vi "PROCESSADOR_bat_PC2.vi"() -> ()   [LabVIEW 2019]
uses:
  <vilib>/Utility/file.llb/Read Delimited Spreadsheet (string).vi
panel:
  out "Numeric":i32
  in  "Previstas":i32=37200
  out "Grupos iter":i32
  out "Freqs iter":i32
  in  "Frequências?":bool=TRUE
  out "Frequência":string
  out "Simulando:":string
  in  "Auto":bool=TRUE
  in  "Ger. Distr.":bool
  in  "Y ? ou D":bool
  in  "Eq. + Trafo":bool=TRUE
  in  "Linhas acopladas":bool=TRUE
  in  "Carga mista":bool=TRUE
  out "path":path
  in  "numera\narquivos":bool
  out "Previstas":i32
  out "Loads (out)":string[](array[string])
  out "inicial":i32
  in  "run minimized? (F)":bool=TRUE
  out "Simulando?":bool
  out "Em processo":i32
  out "Processadas":i32
  out "minutos":dbl
  out "horas":dbl
  out "Elapsed Time (s)":dbl
  in  "Endereço de saída (.atp)":path=path "C:/DADOS/arquivos_atp"
  out "Restantes":i32
  in  "simular?":bool=TRUE
  in  "Endereço de saída (.mat)":path=path "C:/DADOS/Eventos"
  in  "Lista de condições (arquivo.txt)":string="lista_condicoes_CARGAS.txt"
  in  "Diretório de trabalho":path=path "C:/ATP/ATPDraw/Projects_Flavio"
  out "Casos":string[][](array[string])
  # "ATPmanager - Gerenciador de simulações"
  # "*Configurado para operar em conjunto com MATLAB - v2"
  # "Simulações"
  # "________________________________________________________________________"
  # "(trafo com bug - \nusando imped eq)"
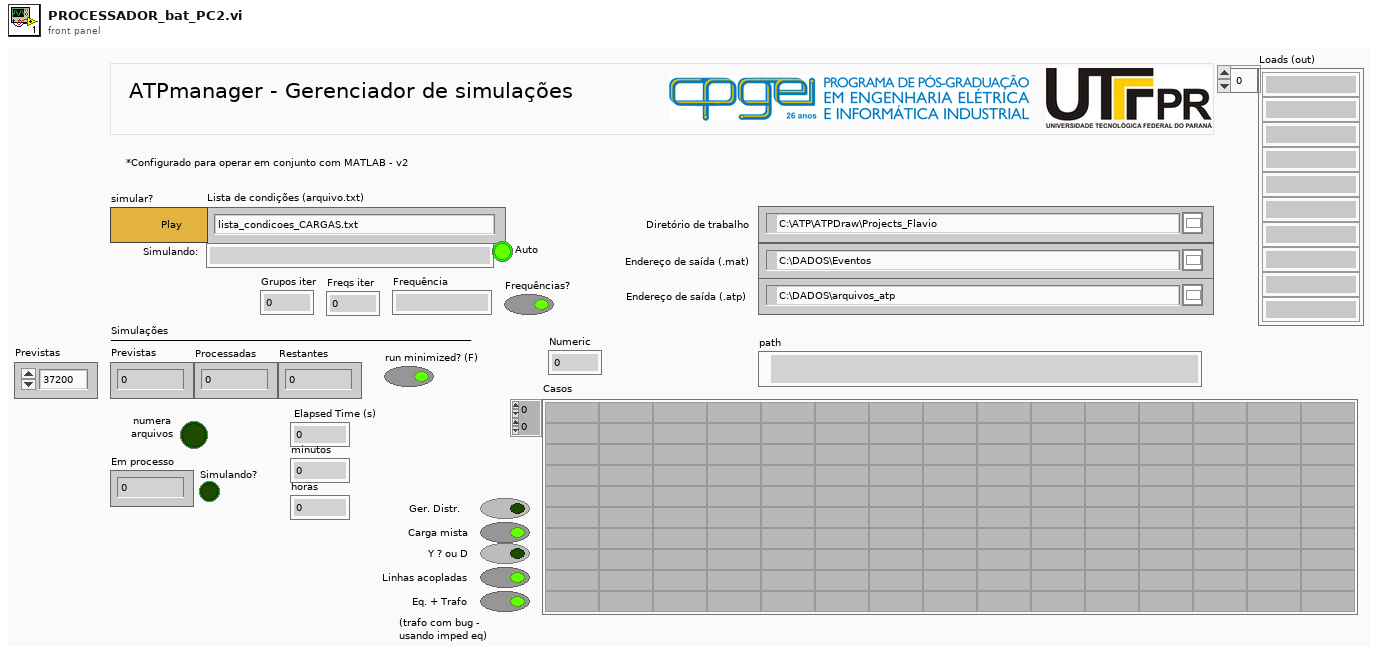
[diagram p1: front panel]
types:
  T1 = cluster{"Ger. Distr.":bool, "Carga mista":bool, "Linhas acopladas":bool, "Eq. + Trafo":bool, "Y ? ou D":bool}
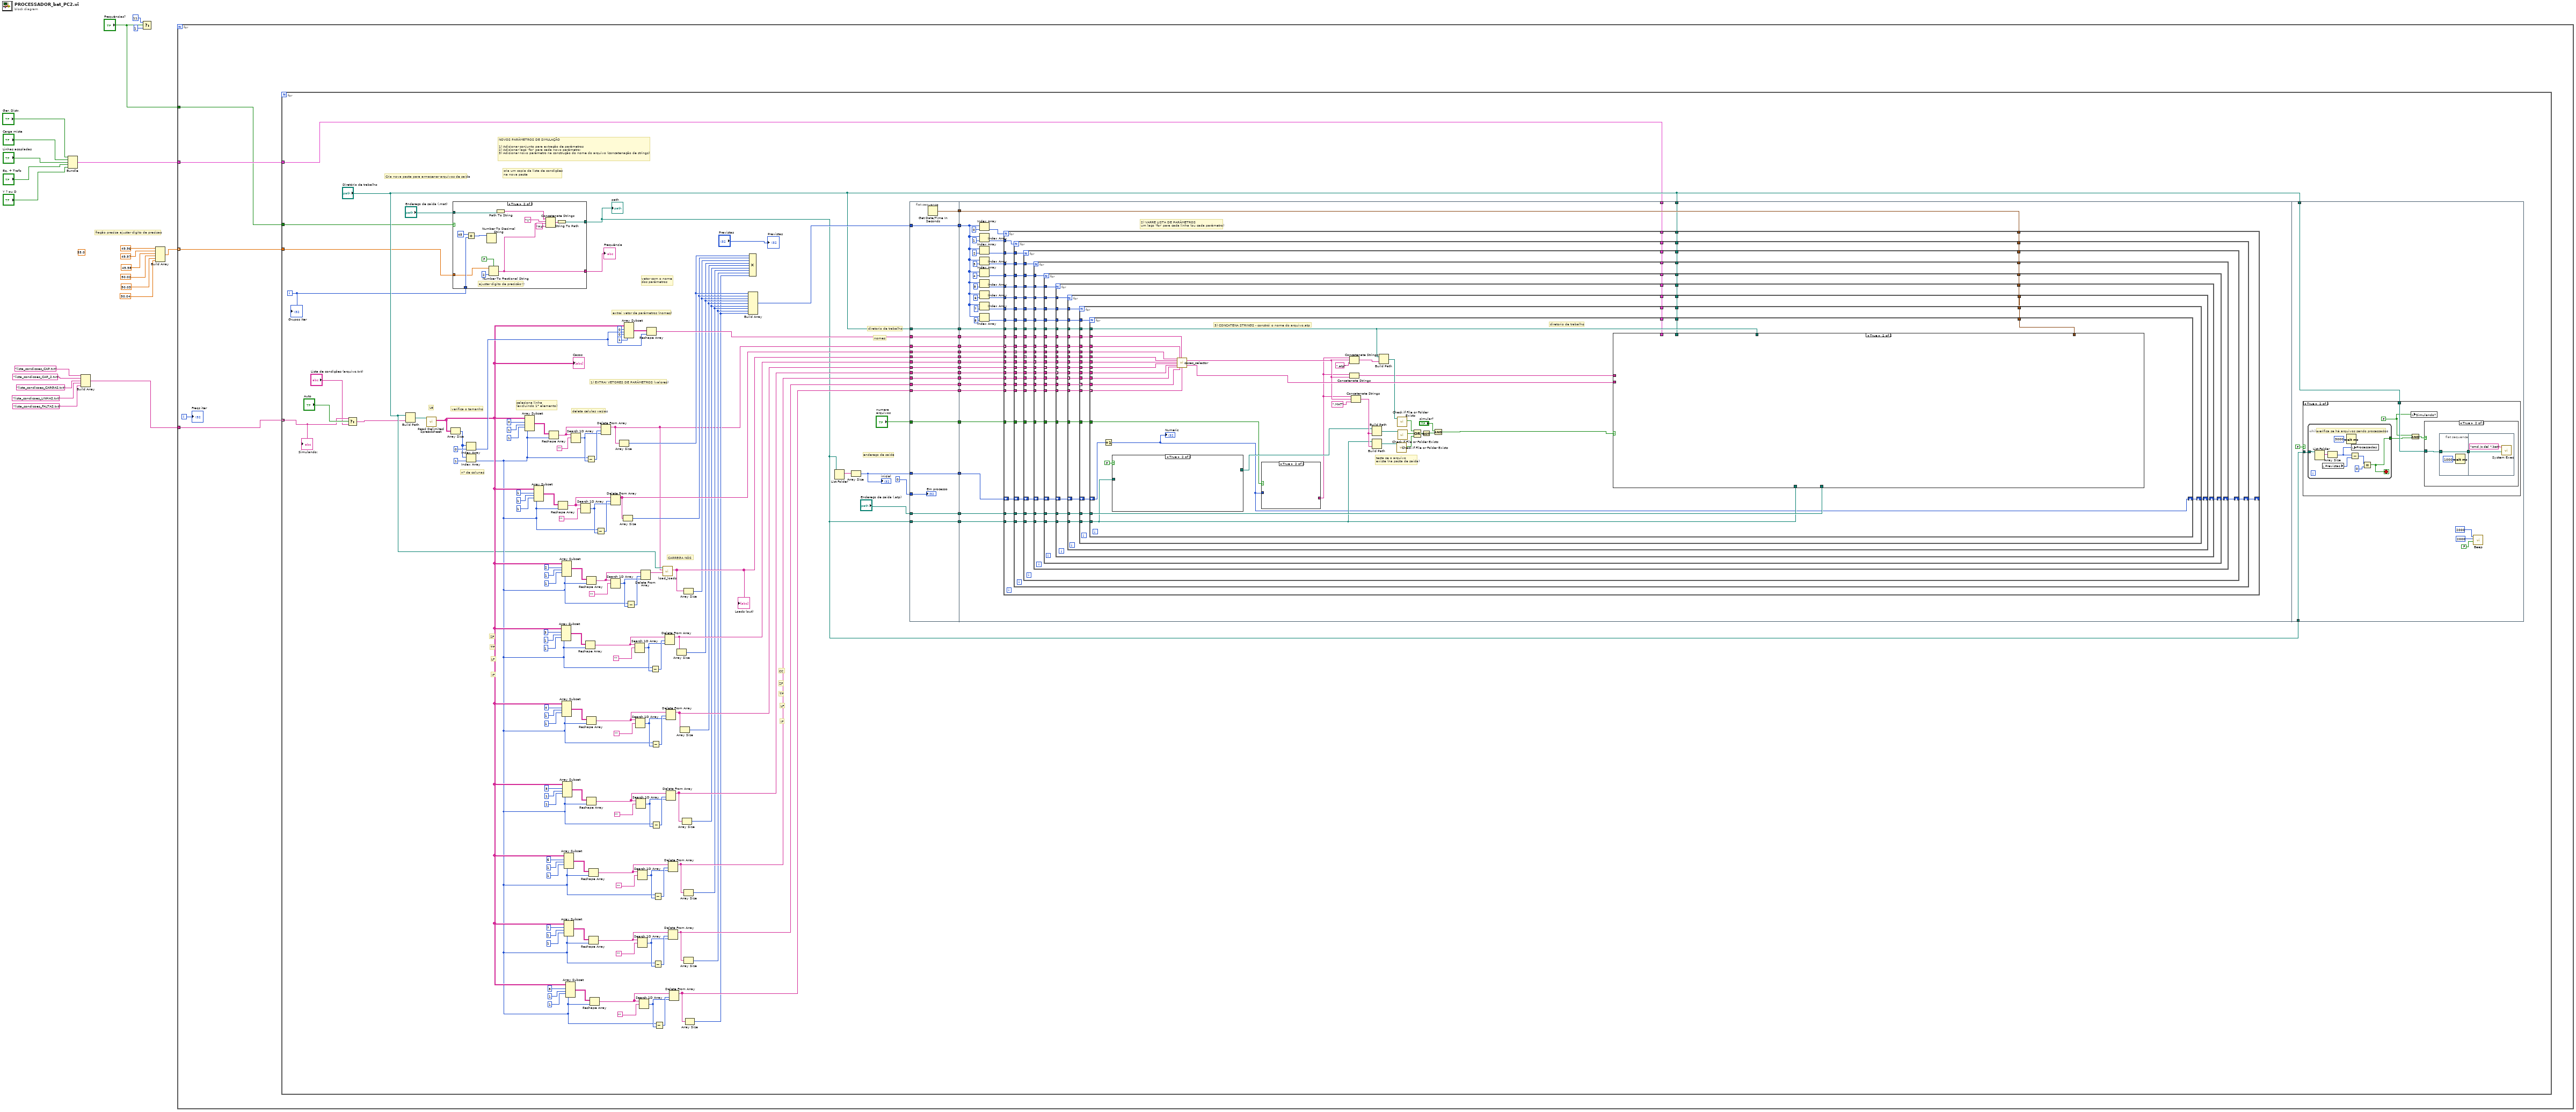
[diagram p0: block diagram]
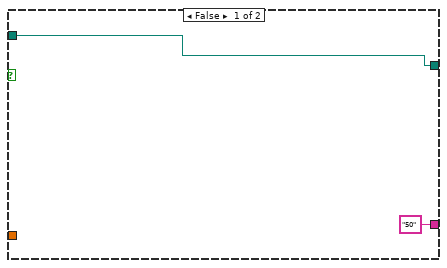
[diagram p2: hidden frame]
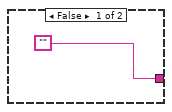
[diagram p4: hidden frame]
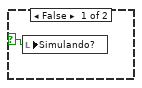
[diagram p5: hidden frame]
diagram:
  (unwired) 55.0
  # "fração precisa ajustar digito de precisao"
  n1 = Bundle("Ger. Distr."="Ger. Distr.", "Carga mista"="Carga mista", "Linhas acopladas"="Linhas acopladas", "Eq. + Trafo"="Eq. + Trafo", "Y ? ou D"="Y ? ou D") -> (w18:T1)  [unwired: 1 in]
  n2 = Build Array("lista_condicoes_CAP.txt", "lista_condicoes_CAP_2.txt", "lista_condicoes_CARGAS.txt", "lista_condicoes_LINHAS.txt", "lista_condicoes_FALTAS.txt") -> (w12:string[])
  n3 = Select(t=11, s="Frequências?", f=1) -> ()  [unwired: 1 out]
  n4 = Build Array(49.96, 49.97, 49.98, 50.02, 50.03, 50.04) -> (w16:dbl[])
  n5 = for {
    tunnel: w18 -> [w27]
    tunnel: w12 -> [w26]
    tunnel: w16 -> [w25] mode=indexing
    tunnel: "Frequências?" -> [w24]
    i -> [w23]
    n6 = for {
      tunnel: w24 -> [w37]
      tunnel: w27 -> [w35]
      tunnel: w26 -> [w32] mode=indexing
      tunnel: w25 -> [w30]
      i -> [w36]
      # "CARREGA NÓS"
      # "deleta celulas vazias"
      # "seleciona linha\n(excluindo 1° elemento)"
      # "endereço de saída"
      # "nomes"
      # "diretorio de trabalho"
      # "LF"
      # "TF"
      # "IF"
      # "ZF"
      # "CC"
      # "LF"
      # "TF"
      # "IF"
      # "ZF"
      # "cria um copia da lista de condições\nna nova pasta"
      # "Cria nova pasta para armazenar arquivos de saída"
      # "extrai vetor de parâmetros (nomes)"
      # "1) EXTRAI VETORES DE PARÂMETROS (valores)"
      # "NOVOS PARÂMETROS DE SIMULAÇÃO\n\n1) Adicionar conjunto para extração de parâmetros\n2) Adicionar laço 'for' para cada novo parâmetro;\n3) Adicionar novo parâmetro na construção do nome do arquivo (concatenação de strings)"
      # "vetor com o nome\ndos parâmetros"
      # "n° de colunas"
      # "verifica o tamanho"
      # "Lê"
      n7 = Select(t=w32, s="Auto", f="Lista de condições (arquivo.txt)") -> (s? t:f=w34:string)
      n8 = Build Path(base path="Diretório de trabalho", name or relative path=w34) -> (appended path=w98:path)
      n9 = call-poly <vilib>:"Read Delimited Spreadsheet.vi"("file path (dialog if empty)"=w98) -> ("all rows"=w59:string[][])  [unwired: 9 in, 5 out]
      "Casos" <- w59
      n10 = Array Size(array=w59) -> (size(s)=w147:i32[])
      n11 = case shown="True" w37 {
        tunnel: [w168 w181] -> w39
        tunnel: "Endereço de saída (.mat)" -> [w168 w179]
        tunnel: w36 -> [_ w175]
        tunnel: w30 -> [_ w170]
        tunnel: ["50" w169] -> w28
        frame False {
        }
        frame True {
          # "ajustar digito de precisão!!!"
          n12 = Add(x=45, y=w175) -> (x+y=w173:i32)
          n13 = Number To Decimal String(number=w173) -> ()  [unwired: 1 in, 1 out]
          n14 = Number To Fractional String(use system decimal point (T)=FALSE, number=w170, precision (6)=i16 2) -> (F-format string=w169:string)  [unwired: 1 in]
          n15 = Path To String(path=w179) -> (string=w178:string)
          n16 = Concatenate Strings(w178, "\\" ("string"), w169, "Hz" ("string")) -> (w180:string)
          n17 = String To Path(string=w180) -> (path=w181:path)
        }
      }
      "path" <- w39
      "Frequência" <- w28
      n18 = Index Array(array=w147, index=0) -> (element=w97:i32)
      n19 = Index Array(array=w147, index=1) -> (element=w58:i32)
      n20 = Array Subset(array=w59, index (row)=0 ("index"), length (row)=1 ("length"), index (col)=1 ("index"), length (col)=w58) -> (w93:string[][])
      n21 = Array Subset(array=w59, index (row)=1 ("index"), length (row)=1 ("length"), index (col)=1 ("index"), length (col)=w58) -> (w139:string[][])
      n22 = Reshape Array(w93, w58) -> (w91:string[])
      n23 = Reshape Array(w139, w58) -> (w137:string[])
      n24 = Array Subset(array=w59, index (row)=3 ("index"), length (row)=1 ("length"), index (col)=1 ("index"), length (col)=w58) -> (w123:string[][])
      n25 = Array Subset(array=w59, index (row)=2 ("index"), length (row)=1 ("length"), index (col)=1 ("index"), length (col)=w58) -> (w131:string[][])
      n26 = Array Subset(array=w59, index (row)=4 ("index"), length (row)=1 ("length"), index (col)=1 ("index"), length (col)=w58) -> (w115:string[][])
      n27 = Array Subset(array=w59, index (row)=5 ("index"), length (row)=1 ("length"), index (col)=1 ("index"), length (col)=w58) -> (w107:string[][])
      n28 = Array Subset(array=w59, index (row)=6 ("index"), length (row)=1 ("length"), index (col)=1 ("index"), length (col)=w58) -> (w80:string[][])
      n29 = Array Subset(array=w59, index (row)=7 ("index"), length (row)=1 ("length"), index (col)=1 ("index"), length (col)=w58) -> (w72:string[][])
      n30 = Array Subset(array=w59, index (row)=8 ("index"), length (row)=1 ("length"), index (col)=1 ("index"), length (col)=w58) -> (w64:string[][])
      n31 = Search 1D Array(1D array=w91, element="") -> (index of element=w89:i32)  [unwired: 1 in]
      n32 = Search 1D Array(1D array=w137, element="") -> (index of element=w135:i32)  [unwired: 1 in]
      n33 = Reshape Array(w123, w58) -> (w121:string[])
      n34 = Subtract(x=w58, y=w89) -> (x-y=w90:i32)
      n35 = Reshape Array(w131, w58) -> (w129:string[])
      n36 = Reshape Array(w115, w58) -> (w113:string[])
      n37 = Reshape Array(w107, w58) -> (w105:string[])
      n38 = Reshape Array(w80, w58) -> (w78:string[])
      n39 = Reshape Array(w72, w58) -> (w70:string[])
      n40 = Reshape Array(w64, w58) -> (w62:string[])
      n41 = Subtract(x=w58, y=w135) -> (x-y=w136:i32)
      n42 = Delete From Array(array=w91, length=w90, index=w89) -> (array with subset deleted=w41:string[])  [unwired: 1 out]
      n43 = Delete From Array(array=w137, length=w136, index=w135) -> (array with subset deleted=w87:string[])  [unwired: 1 out]
      n44 = Search 1D Array(1D array=w129, element="") -> (index of element=w127:i32)  [unwired: 1 in]
      n45 = Array Size(array=w41) -> (size(s)=w50:i32)
      n46 = Array Size(array=w87) -> (size(s)=w49:i32)
      n47 = Array Subset(array=w59, index (row)=0 ("index"), length (row)=w97, index (col)=0 ("index"), length (col)=1 ("length")) -> (w143:string[][])
      n48 = Subtract(x=w58, y=w127) -> (x-y=w128:i32)
      n49 = Search 1D Array(1D array=w121, element="") -> (index of element=w119:i32)  [unwired: 1 in]
      n50 = Search 1D Array(1D array=w113, element="") -> (index of element=w111:i32)  [unwired: 1 in]
      n51 = Search 1D Array(1D array=w105, element="") -> (index of element=w103:i32)  [unwired: 1 in]
      n52 = Search 1D Array(1D array=w78, element="") -> (index of element=w76:i32)  [unwired: 1 in]
      n53 = Search 1D Array(1D array=w70, element="") -> (index of element=w68:i32)  [unwired: 1 in]
      n54 = Search 1D Array(1D array=w62, element="") -> (index of element=w60:i32)  [unwired: 1 in]
      n55 = Delete From Array(array=w129, length=w128, index=w127) -> (array with subset deleted=w53:string[])  [unwired: 1 out]
      n56 = Reshape Array(w143, w97) -> (w96:string[])
      n57 = Subtract(x=w58, y=w119) -> (x-y=w120:i32)
      n58 = Subtract(x=w58, y=w111) -> (x-y=w112:i32)
      n59 = Subtract(x=w58, y=w103) -> (x-y=w104:i32)
      n60 = Subtract(x=w58, y=w76) -> (x-y=w77:i32)
      n61 = Subtract(x=w58, y=w68) -> (x-y=w69:i32)
      n62 = Subtract(x=w58, y=w60) -> (x-y=w61:i32)
      n63 = call "load_loads.vi"("Nodes"=w53, "Events"=w41, "Diretório de trabalho"="Diretório de trabalho") -> ("Loads (out)"=w51:string[])  [unwired: 8 in]
      "Loads (out)" <- w51
      n64 = Delete From Array(array=w121, length=w120, index=w119) -> (array with subset deleted=w86:string[])  [unwired: 1 out]
      n65 = Delete From Array(array=w113, length=w112, index=w111) -> (array with subset deleted=w85:string[])  [unwired: 1 out]
      n66 = Delete From Array(array=w105, length=w104, index=w103) -> (array with subset deleted=w84:string[])  [unwired: 1 out]
      n67 = Delete From Array(array=w78, length=w77, index=w76) -> (array with subset deleted=w57:string[])  [unwired: 1 out]
      n68 = Delete From Array(array=w70, length=w69, index=w68) -> (array with subset deleted=w56:string[])  [unwired: 1 out]
      n69 = Delete From Array(array=w62, length=w61, index=w60) -> (array with subset deleted=w55:string[])  [unwired: 1 out]
      n70 = Array Size(array=w86) -> (size(s)=w47:i32)
      n71 = Array Size(array=w85) -> (size(s)=w46:i32)
      n72 = Array Size(array=w84) -> (size(s)=w45:i32)
      n73 = Array Size(array=w51) -> (size(s)=w48:i32)
      n74 = Array Size(array=w57) -> (size(s)=w44:i32)
      n75 = Array Size(array=w56) -> (size(s)=w43:i32)
      n76 = Array Size(array=w55) -> (size(s)=w42:i32)
      n77 = Build Array(w50, w49, w48, w47, w46, w45, w44, w43, w42) -> (w54:i32[])
      n78 = Compound Arithmetic op=MULTIPLY(w50, w49, w48, w47, w46, w45, w44, w43, w42) -> ()  [unwired: 1 out]
      n79 = List Folder(path=w39) -> (filenames=w100:string[])  [unwired: 3 in, 3 out]
      n80 = Array Size(array=w100) -> (size(s)=w99:i32)
      "inicial" <- w99
      n81 = flat-sequence {
        tunnel: w96 -> [w198]
        tunnel: "Diretório de trabalho" -> [w199]
        tunnel: [w199] -> w166
        tunnel: [w198] -> w165
        tunnel: [w197] -> w164
        tunnel: "Endereço de saída (.atp)" -> [w197]
        tunnel: [w196] -> w163
        tunnel: [w193] -> w162
        tunnel: 0 -> [w195]
        tunnel: w39 -> [w194]
        tunnel: [w194] -> w161
        tunnel: w99 -> [w193]
        tunnel: w54 -> [w192]
        tunnel: [w192] -> w160
        tunnel: w41 -> [w191]
        tunnel: [w191] -> w159
        tunnel: w87 -> [w190]
        tunnel: w51 -> [w189]
        tunnel: w86 -> [w188]
        tunnel: w85 -> [w187]
        tunnel: w84 -> [w186]
        tunnel: [w190] -> w158
        tunnel: [w189] -> w157
        tunnel: [w188] -> w156
        tunnel: [w187] -> w155
        tunnel: [w186] -> w154
        tunnel: [w185] -> w153
        tunnel: w57 -> [w185]
        tunnel: [w184] -> w152
        tunnel: w56 -> [w184]
        tunnel: [w183] -> w151
        tunnel: w55 -> [w183]
        tunnel: [w182] -> w150
        tunnel: "numera\narquivos" -> [w182]
        tunnel: w166 -> [w236]
        tunnel: w165 -> [w235]
        tunnel: w164 -> [w234]
        tunnel: w163 -> [w233]
        tunnel: w162 -> [w230]
        tunnel: w161 -> [w232]
        tunnel: "Diretório de trabalho" -> [w231]
        tunnel: w160 -> [w220]
        tunnel: w159 -> [w210]
        tunnel: w158 -> [w209]
        tunnel: w157 -> [w208]
        tunnel: w156 -> [w207]
        tunnel: w155 -> [w206]
        tunnel: w154 -> [w205]
        tunnel: w153 -> [w204]
        tunnel: w152 -> [w203]
        tunnel: w151 -> [w202]
        tunnel: w150 -> [w201]
        tunnel: w35 -> [w200]
        tunnel: "Diretório de trabalho" -> [w540]
        tunnel: w39 -> [w541]
        frame #0 {
          n82 = Get Date/Time In Seconds() -> (seconds since 1Jan1904=w196:timestamp)
          "Em processo" <- w195
        }
        frame #1 {
          # "2) VARRE LISTA DE PARÂMETROS\num laço 'for' para cada linha (ou cada parâmetro)"
          n83 = Index Array(array=w220, index=0) -> (element=w219:i32)
          n84 = Index Array(array=w220, index=1) -> (element=w218:i32)
          n85 = Index Array(array=w220, index=2) -> (element=w217:i32)
          n86 = Index Array(array=w220, index=3) -> (element=w216:i32)
          n87 = Index Array(array=w220, index=4) -> (element=w215:i32)
          n88 = Index Array(array=w220, index=5) -> (element=w214:i32)
          n89 = Index Array(array=w220, index=6) -> (element=w213:i32)
          n90 = Index Array(array=w220, index=7) -> (element=w212:i32)
          n91 = Index Array(array=w220, index=8) -> (element=w211:i32)
          n92 = for {
            N: w219 -> [_]
            tunnel: w236 -> [w263]
            tunnel: w235 -> [w262]
            tunnel: w234 -> [w261]
            tunnel: w233 -> [w260]
            tunnel: w232 -> [w258]
            tunnel: w231 -> [w257]
            shift-right: [w259] -> _
            shift-left: w230 -> [w256]
            tunnel: w218 -> [w255]
            tunnel: w217 -> [w254]
            tunnel: w216 -> [w253]
            tunnel: w215 -> [w252]
            tunnel: w214 -> [w251]
            tunnel: w213 -> [w250]
            tunnel: w212 -> [w249]
            tunnel: w211 -> [w248]
            tunnel: w210 -> [w247] mode=indexing
            tunnel: w209 -> [w246]
            tunnel: w208 -> [w245]
            tunnel: w207 -> [w244]
            tunnel: w206 -> [w243]
            tunnel: w205 -> [w242]
            tunnel: w204 -> [w241]
            tunnel: w203 -> [w240]
            tunnel: w202 -> [w239]
            tunnel: w201 -> [w238]
            tunnel: w200 -> [w237]
            n93 = for {
              N: w255 -> [_]
              tunnel: w263 -> [w289]
              tunnel: w262 -> [w288]
              tunnel: w261 -> [w287]
              tunnel: w260 -> [w286]
              tunnel: w258 -> [w284]
              tunnel: w257 -> [w283]
              shift-right: [w285] -> w259
              shift-left: w256 -> [w282]
              tunnel: w254 -> [w281]
              tunnel: w253 -> [w280]
              tunnel: w252 -> [w279]
              tunnel: w251 -> [w278]
              tunnel: w250 -> [w277]
              tunnel: w249 -> [w276]
              tunnel: w248 -> [w275]
              tunnel: w247 -> [w274]
              tunnel: w246 -> [w273] mode=indexing
              tunnel: w245 -> [w272]
              tunnel: w244 -> [w271]
              tunnel: w243 -> [w270]
              tunnel: w242 -> [w269]
              tunnel: w241 -> [w268]
              tunnel: w240 -> [w267]
              tunnel: w239 -> [w266]
              tunnel: w238 -> [w265]
              tunnel: w237 -> [w264]
              n94 = for {
                N: w281 -> [_]
                tunnel: w289 -> [w314]
                tunnel: w288 -> [w313]
                tunnel: w287 -> [w312]
                tunnel: w286 -> [w311]
                tunnel: w284 -> [w309]
                tunnel: w283 -> [w308]
                shift-right: [w310] -> w285
                shift-left: w282 -> [w307]
                tunnel: w280 -> [w306]
                tunnel: w279 -> [w305]
                tunnel: w278 -> [w304]
                tunnel: w277 -> [w303]
                tunnel: w276 -> [w302]
                tunnel: w275 -> [w301]
                tunnel: w274 -> [w300]
                tunnel: w273 -> [w299]
                tunnel: w272 -> [w298] mode=indexing
                tunnel: w271 -> [w297]
                tunnel: w270 -> [w296]
                tunnel: w269 -> [w295]
                tunnel: w268 -> [w294]
                tunnel: w267 -> [w293]
                tunnel: w266 -> [w292]
                tunnel: w265 -> [w291]
                tunnel: w264 -> [w290]
                n95 = for {
                  N: w306 -> [_]
                  tunnel: w314 -> [w338]
                  tunnel: w313 -> [w337]
                  shift-right: [w336] -> w310
                  shift-left: w307 -> [w333]
                  tunnel: w312 -> [w335]
                  tunnel: w311 -> [w334]
                  tunnel: w309 -> [w332]
                  tunnel: w308 -> [w331]
                  tunnel: w305 -> [w329]
                  tunnel: w304 -> [w330]
                  tunnel: w303 -> [w328]
                  tunnel: w302 -> [w327]
                  tunnel: w301 -> [w326]
                  tunnel: w300 -> [w325]
                  tunnel: w299 -> [w324]
                  tunnel: w298 -> [w323]
                  tunnel: w297 -> [w322] mode=indexing
                  tunnel: w296 -> [w321]
                  tunnel: w295 -> [w320]
                  tunnel: w294 -> [w319]
                  tunnel: w293 -> [w318]
                  tunnel: w292 -> [w317]
                  tunnel: w291 -> [w316]
                  tunnel: w290 -> [w315]
                  n96 = for {
                    N: w329 -> [_]
                    tunnel: w337 -> [w361]
                    tunnel: w338 -> [w360]
                    shift-right: [w358] -> w336
                    shift-left: w333 -> [w359]
                    tunnel: w335 -> [w357]
                    tunnel: w334 -> [w356]
                    tunnel: w332 -> [w355]
                    tunnel: w331 -> [w354]
                    tunnel: w330 -> [w353]
                    tunnel: w328 -> [w352]
                    tunnel: w327 -> [w351]
                    tunnel: w326 -> [w350]
                    tunnel: w325 -> [w349]
                    tunnel: w324 -> [w348]
                    tunnel: w323 -> [w347]
                    tunnel: w322 -> [w346]
                    tunnel: w321 -> [w344] mode=indexing
                    tunnel: w320 -> [w345]
                    tunnel: w319 -> [w343]
                    tunnel: w318 -> [w342]
                    tunnel: w317 -> [w341]
                    tunnel: w316 -> [w340]
                    tunnel: w315 -> [w339]
                    n97 = for {
                      N: w353 -> [_]
                      tunnel: w361 -> [w383]
                      tunnel: w360 -> [w382]
                      shift-right: [w380] -> w358
                      shift-left: w359 -> [w381]
                      tunnel: w357 -> [w379]
                      tunnel: w356 -> [w378]
                      tunnel: w355 -> [w377]
                      tunnel: w354 -> [w376]
                      tunnel: w352 -> [w375]
                      tunnel: w351 -> [w374]
                      tunnel: w350 -> [w373]
                      tunnel: w349 -> [w372]
                      tunnel: w348 -> [w371]
                      tunnel: w347 -> [w370]
                      tunnel: w346 -> [w369]
                      tunnel: w345 -> [w368] mode=indexing
                      tunnel: w344 -> [w367]
                      tunnel: w343 -> [w366]
                      tunnel: w342 -> [w365]
                      tunnel: w341 -> [w364]
                      tunnel: w340 -> [w363]
                      tunnel: w339 -> [w362]
                      n98 = for {
                        N: w375 -> [_]
                        tunnel: w383 -> [w404]
                        tunnel: w382 -> [w403]
                        shift-right: [w401] -> w380
                        shift-left: w381 -> [w402]
                        tunnel: w379 -> [w400]
                        tunnel: w378 -> [w399]
                        tunnel: w377 -> [w398]
                        tunnel: w376 -> [w397]
                        tunnel: w374 -> [w396]
                        tunnel: w373 -> [w395]
                        tunnel: w372 -> [w394]
                        tunnel: w371 -> [w393]
                        tunnel: w370 -> [w392]
                        tunnel: w369 -> [w391]
                        tunnel: w368 -> [w390]
                        tunnel: w367 -> [w389]
                        tunnel: w366 -> [w388] mode=indexing
                        tunnel: w365 -> [w387]
                        tunnel: w364 -> [w386]
                        tunnel: w363 -> [w385]
                        tunnel: w362 -> [w384]
                        n99 = for {
                          N: w396 -> [_]
                          tunnel: w404 -> [w424]
                          tunnel: w403 -> [w423]
                          shift-right: [w421] -> w401
                          shift-left: w402 -> [w422]
                          tunnel: w400 -> [w420]
                          tunnel: w399 -> [w419]
                          tunnel: w398 -> [w418]
                          tunnel: w397 -> [w417]
                          tunnel: w395 -> [w416]
                          tunnel: w394 -> [w415]
                          tunnel: w393 -> [w414]
                          tunnel: w392 -> [w413]
                          tunnel: w391 -> [w412]
                          tunnel: w390 -> [w411]
                          tunnel: w389 -> [w410]
                          tunnel: w388 -> [w409]
                          tunnel: w387 -> [w408] mode=indexing
                          tunnel: w386 -> [w407]
                          tunnel: w385 -> [w406]
                          tunnel: w384 -> [w405]
                          n100 = for {
                            N: w416 -> [_]
                            tunnel: w424 -> [w447]
                            tunnel: w423 -> [w462]
                            shift-right: [w425] -> w421
                            shift-left: w422 -> [w427]
                            tunnel: w420 -> [w461]
                            tunnel: w419 -> [w460]
                            tunnel: w418 -> [w434]
                            tunnel: w417 -> [w449]
                            tunnel: w415 -> [w446]
                            tunnel: w414 -> [w445]
                            tunnel: w413 -> [w444]
                            tunnel: w412 -> [w443]
                            tunnel: w411 -> [w441]
                            tunnel: w410 -> [w442]
                            tunnel: w409 -> [w440]
                            tunnel: w408 -> [w439]
                            tunnel: w407 -> [w438] mode=indexing
                            tunnel: w406 -> [w432]
                            tunnel: w405 -> [w428]
                            # "diretorio de trabalho"
                            # "testa se o arquivo\nexiste (na pasta de saída)"
                            # "3) CONCATENA STRINGS - constrói o nome do arquivo.atp"
                            n101 = Increment(x=w427) -> (x+1=w425:i32)
                            "Numeric" <- w425
                            n102 = case shown="True" FALSE {
                              tunnel: [w464 w466] -> w435
                              tunnel: w434 -> [w464 w465]
                              frame False {
                              }
                              frame True {
                                n103 = flat-sequence {
                                tunnel: w465 -> [w469]
                                tunnel: [w470] -> w468
                                tunnel: [w469] -> w467
                                tunnel: [w472] -> w466
                                tunnel: w468 -> [w473]
                                tunnel: w467 -> [w472]
                                frame #0 {
                                n104 = List Folder(path=w469) -> (filenames=w471:string[])  [unwired: 3 in, 3 out]
                                n105 = Array Size(array=w471) -> (size(s)=w470:i32)
                                "Processadas" <- w470
                                }
                                frame #1 {
                                n106 = local read "Previstas"() -> (w474:i32)
                                n107 = Subtract(x=w474, y=w473) -> (x-y=→"Restantes":i32)
                                }
                                }
                              }
                            }
                            n108 = call "cases_selector.vi"("Q - quantidade (p.u.)"=w445, "N - nó"=w444, "C - condição de carga (p.u.)"=w443, "Z - impedância de falta (Ohms)"=w442, "I - instante de falta (ms)"=w441, "L - local de falta"=w440, "E - evento"=w446, "T - tipo de falta"=w439, "Parâmetros"=w447, "M - mecânica"=w438) -> ("nome do arquivo"=w431:string, "dados"=w437:string[])  [unwired: 8 in]
                            n109 = case shown="True" w432 {
                              tunnel: w425 -> [_ w479]
                              tunnel: ["" w480] -> w429
                              frame False {
                              }
                              frame True {
                                n110 = Add(x=0, y=w479) -> (x+y=w477:i32)
                                n111 = call "Build Text"("number"=w477) -> ("Result"=w480:string)  [unwired: 13 in, 1 out]
                              }
                            }
                            n112 = Concatenate Strings(w429, w431, ".atp") -> (w452:string)
                            n113 = Concatenate Strings(w429, w431) -> (w430:string)
                            n114 = Concatenate Strings(w429, w431, ".MAT" ("string")) -> (w450:string)
                            n115 = Build Path(base path=w435, name or relative path=w450) -> (appended path=w463:path)
                            n116 = Build Path(base path=w434, name or relative path=w450) -> (appended path=w453:path)
                            n117 = Build Path(base path=w462, name or relative path=w452) -> (appended path=w436:path)
                            n118 = call <vilib>:"Check if File or Folder Exists.vi"("path"=w453) -> ("file or folder exists?"=w454:bool)  [unwired: 8 in, 2 out]
                            n119 = call <vilib>:"Check if File or Folder Exists.vi"("path"=w436) -> ("file or folder exists?"=w456:bool)  [unwired: 8 in, 2 out]
                            n120 = call <vilib>:"Check if File or Folder Exists.vi"("path"=w463) -> ("file or folder exists?"=w455:bool)  [unwired: 8 in, 2 out]
                            n121 = Compound Arithmetic op=OR(w456, w455, w454) -> (w457:bool)
                            n122 = Not(x=w457) -> (.not. x?=w459:bool)
                            n123 = Compound Arithmetic op=AND("simular?", w459) -> (w433:bool)
                            n124 = case shown="True" w433 {
                              selector: w433 -> [w481 w489]
                              tunnel: w462 -> [_ w483]
                              tunnel: w430 -> [_ w499]
                              tunnel: w434 -> [_ w496]
                              tunnel: w461 -> [_ w492]
                              tunnel: w460 -> [_ w491]
                              tunnel: w449 -> [_ w487]
                              tunnel: w437 -> [_ w486]
                              tunnel: w428 -> [_ w482]
                              frame False {
                                n125 = local write "Simulando?"(w481) -> ()
                              }
                              frame True {
                                n126 = flat-sequence {
                                tunnel: [w505] -> w495
                                tunnel: w499 -> [w505]
                                tunnel: [w504] -> w493
                                tunnel: w487 -> [w502]
                                tunnel: w486 -> [w503]
                                tunnel: w482 -> [w501]
                                tunnel: w495 -> [w507]
                                tunnel: [w507] -> w494
                                tunnel: w493 -> [_]
                                tunnel: w494 -> [w510]
                                tunnel: [w518] -> w498
                                tunnel: w483 -> [w514]
                                tunnel: [w516] -> w497
                                tunnel: w496 -> [w508]
                                tunnel: w492 -> [w512]
                                tunnel: [w510] -> w490
                                tunnel: [w508] -> w484
                                tunnel: w483 -> [w528]
                                tunnel: w498 -> [w527]
                                tunnel: w497 -> [w526]
                                tunnel: [w522] -> w488
                                tunnel: w490 -> [_]
                                tunnel: [w520] -> w485
                                tunnel: w484 -> [w520]
                                tunnel: w491 -> [_]
                                tunnel: w488 -> [_]
                                tunnel: w485 -> [w529]
                                tunnel: w483 -> [w530]
                                frame #0 {
                                # "constroi .atp"
                                n127 = local read "Frequência"() -> (w500:string)
                                n128 = call "constroi_atp.vi"("archive name"=w505, "directory out"=w502, "dados"=w503, "Parâmetros"=w501, "Frequência"=w500) -> ("concatenated string"=w504:string)  [unwired: 10 in]
                                }
                                frame #1 {
                                n129 = Wait (ms)(milliseconds to wait=u32 150) -> ()  [unwired: 1 out]
                                }
                                frame #2 {
                                # "constroi .bat"
                                n130 = Path To String(path=w514) -> (string=w515:string)
                                n131 = Concatenate Strings(w510, ".bat" ("string")) -> (w516:string)
                                n132 = Path To String(path=w508) -> (string=w513:string)
                                n133 = Path To String(path=w512) -> (string=w511:string)
                                n134 = Build Path(base path=w514, name or relative path=w516) -> (appended path=w517:path)
                                n135 = call "ALTERA_BAT.vi"("file path (use dialog)"=w517, "Diretório de trabalho (.atp)"=w515, "Nome do arquivo"=w510, "Diretório de saída"=w513, "Diretório de saída (arquivos atp)"=w511) -> ("error out"=w518:errorcluster)  [unwired: 9 in, 1 out]
                                }
                                frame #3 {
                                # "manda executar .bat"
                                # "converte .pl4 -> .mat"
                                n136 = Concatenate Strings("cmd /c " ("string"), w526) -> (w524:string)
                                n137 = call <vilib>:"System Exec.vi"("expected output size  (4096)"=u32 65536, "run minimized? (F)"="run minimized? (F)", "wait until completion? (T)"=TRUE, "error in (no error)"=w527, "working directory"=w528, "command line"=w524) -> ("error out"=w522:errorcluster)  [unwired: 2 in, 3 out]
                                }
                                frame #4 {
                                n138 = call "Elapsed Time"() -> ("Elapsed Time (s)"=w531:dbl)  [unwired: 12 in, 7 out]
                                "Elapsed Time (s)" <- w531
                                n139 = Divide(x=w531, y=60.0) -> (x/y=w534:dbl)
                                "minutos" <- w534
                                n140 = Divide(x=w534, y=60.0) -> (x/y=→"horas":dbl)
                                n141 = call "del_bats.vi"("Endereço de saída (.mat)"=w529, "Diretório de trabalho"=w530) -> ()  [unwired: 10 in]
                                }
                                }
                                "Simulando?" <- w489
                              }
                            }
                          }
                        }
                      }
                    }
                  }
                }
              }
            }
          }
        }
        frame #2 {
          n142 = case shown="True" FALSE {
            tunnel: w541 -> [_ w546]
            tunnel: w540 -> [_ w545]
            frame False {
            }
            frame True {
              w542 = FALSE ("x")
              n143 = while {
                tunnel: w546 -> [w560]
                tunnel: [w557] -> w544
                stop <- w557 stop-if-true
                # "verifica se há arquivos sendo processados"
                n144 = List Folder(path=w560) -> (filenames=w559:string[])  [unwired: 3 in, 3 out]
                n145 = local read "Previstas"() -> (w555:i32)
                n146 = Array Size(array=w559) -> (size(s)=w553:i32)
                n147 = Wait (ms)(milliseconds to wait=u32 3000) -> ()  [unwired: 1 out]
                n148 = Subtract(x=w553, y=w555) -> (x-y=w554:i32)
                n149 = local write "Processadas"(w553) -> ()
                n150 = Equal?(x=w554, y=0) -> (x = y?=w557:bool)
              }
              n151 = And(x=w542, y=w544) -> (x .and. y?=w543:bool)
              n152 = local write "Simulando?"(w542) -> ()
              n153 = case shown="True" w543 {
                tunnel: w545 -> [_ w548]
                frame False {
                }
                frame True {
                  n154 = flat-sequence {
                    tunnel: w548 -> [w550]
                    tunnel: [w550] -> w547
                    tunnel: w547 -> [w551]
                    frame #0 {
                      n155 = Wait (ms)(milliseconds to wait=u32 1000) -> ()  [unwired: 1 out]
                    }
                    frame #1 {
                      n156 = call <vilib>:"System Exec.vi"("working directory"=w551, "command line"="cmd /c del *.bat") -> ()  [unwired: 6 in, 4 out]
                    }
                  }
                }
              }
            }
          }
          n157 = call <vilib>:"Beep.vi"("use system alert? (T)"=FALSE, "duration (msec)"=u32 2000, "frequency (Hz)"=u32 2000) -> ()  [unwired: 9 in]
        }
      }
      "Previstas" <- "Previstas"
      "Simulando:" <- w32
      "Grupos iter" <- w36
    }
    "Freqs iter" <- w23
  }
